vi "Swap DDS and CS.vi"(6 "Variant in":variant, 7 "Shift Pressed?":bool, 8 "error in (no error)":errorcluster, 10 "QD Combo Box Ref":refnum<vi>, 11 "QD Launch VI Ref":refnum<vi>) -> (0 "error out":errorcluster, 4 "Variant out":variant)   [LabVIEW 2017]
doc: "This VI is almost the same as \"Insert or Replace.vi\" QuickDrop shortcut by Darren Nattinger (https://forums.ni.com/t5/Quick-Drop-Enthusiasts/Quick-Drop-Keyboard-Shortcut-Replace-or-Insert/gpm-p/3534994?profile.language=en). It just calls \"Insert From Clipboard.vi\" and \"Replace From Clipboard.vi\" by Tritem instead of LabVIEW default ones.\n\nDefault Shortcut - [H]"
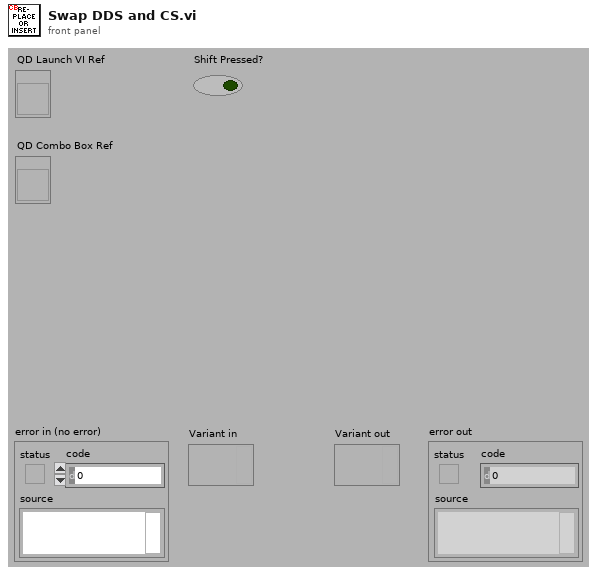
[diagram p1: front panel]
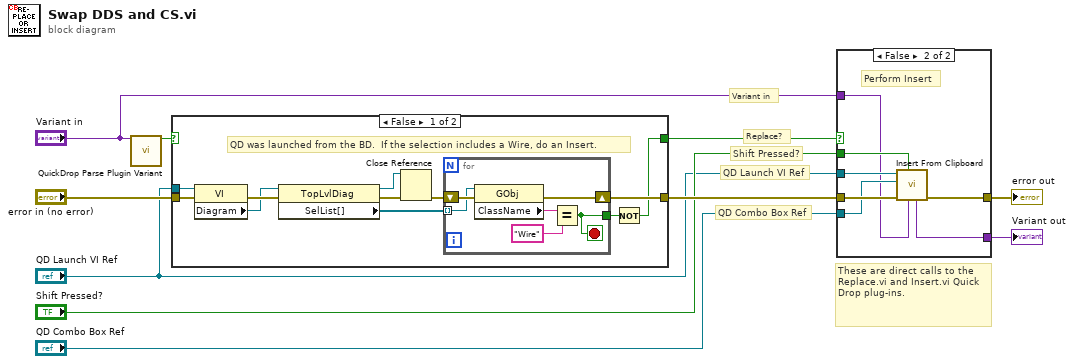
[diagram p0: block diagram]
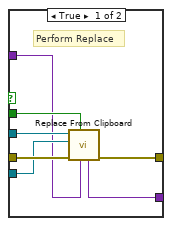
[diagram p2: hidden frame]
diagram:
  # "Replace?"
  # "Variant in"
  # "Shift Pressed?"
  # "QD Launch VI Ref"
  # "QD Combo Box Ref"
  # "These are direct calls to the Replace.vi and Insert.vi Quick Drop plug-ins."
  n1 = call <vilib>:"QuickDrop Parse Plugin Variant.vi"("QDKS Variant in"="Variant in") -> ("QD Launch VI Panel?"=w9:bool)  [unwired: 12 in, 2 out]
  n2 = case shown="False" w9 {
    selector: w9 -> [_ w29]
    tunnel: "error in (no error)" -> [w19 w28]
    tunnel: "QD Launch VI Ref" -> [w18 _]
    tunnel: [w17 w28] -> w7
    tunnel: [w11 w29] -> w8
    frame False {
      # "QD was launched from the BD.  If the selection includes a Wire, do an Insert."
      n3 = property class="VI"(reference=w18, error in=w19) -> (error out=w16:errorcluster, "Diagram"=w15:refnum<vi>)  [unwired: 1 out]
      n4 = property class="TopLvlDiag"(reference=w15, error in=w16) -> (reference out=w13:refnum<vi>, error out=w14:errorcluster, "SelList[]"=w20:refnum<vi>[])
      n5 = Close Reference(reference=w13, error in (no error)=w14) -> (error out=w21:errorcluster)
      n6 = for {
        shift-right: [w26] -> w17
        shift-left: w21 -> [w27]
        tunnel: w20 -> [w25] mode=indexing
        tunnel: [w22] -> w12
        stop <- w22 stop-if-true
        n7 = property class="GObj"(reference=w25, error in=w27) -> (error out=w26:errorcluster, "ClassName"=w24:string)  [unwired: 1 out]
        n8 = Equal?(x=w24, y="Wire") -> (x = y?=w22:bool)
      }
      n9 = Not(x=w12) -> (.not. x?=w11:bool)
    }
    frame True {
      # "QD was launched from the panel.  This must be a Replace."
    }
  }
  n10 = case shown="False" w8 {
    tunnel: w7 -> [w36 w43]
    tunnel: [w35 w42] -> w6
    tunnel: "Variant in" -> [w30 w37]
    tunnel: "Shift Pressed?" -> [w34 w41]
    tunnel: "QD Launch VI Ref" -> [w33 w40]
    tunnel: "QD Combo Box Ref" -> [w32 w39]
    tunnel: [w31 w38] -> w1
    frame True {
      # "Perform Replace"
      n11 = call <resource>:"Replace From Clipboard.vi"("Variant in"=w30, "Shift Pressed?"=w34, "error in (no error)"=w36, "QD Combo Box Ref"=w32, "QD Launch VI Ref"=w33) -> ("error out"=w35:errorcluster, "Variant out"=w31:variant)  [unwired: 5 in]
    }
    frame False {
      # "Perform Insert"
      n12 = call <resource>:"Insert From Clipboard.vi"("Variant in"=w37, "Shift Pressed?"=w41, "error in (no error)"=w43, "QD Combo Box Ref"=w39, "QD Launch VI Ref"=w40) -> ("error out"=w42:errorcluster, "Variant out"=w38:variant)  [unwired: 5 in]
    }
  }
  "error out" <- w6
  "Variant out" <- w1
